vi "mudança cores.vi"() -> ()   [LabVIEW 2018]
panel:
  in  "stop":bool
  out "Thermometer":dbl(slide) scale=0.0..100.0
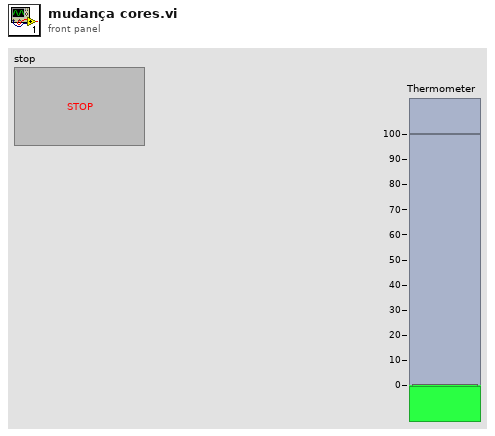
[diagram p1: front panel]
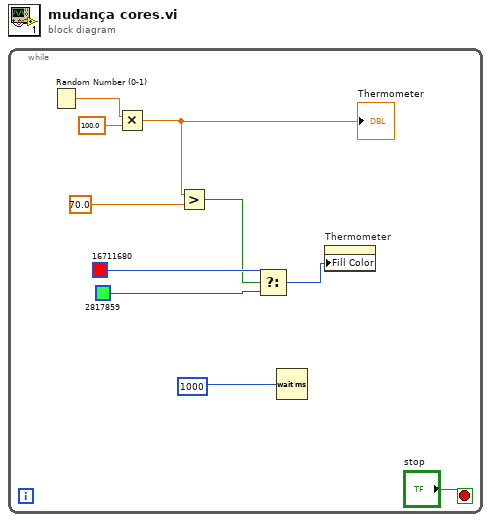
[diagram p0: block diagram]
diagram:
  n1 = while {
    stop <- "stop" stop-if-true
    n2 = Random Number (0-1)() -> (number: 0 to 1=w9:dbl)
    n3 = Multiply(x=w9, y=100.0) -> (x*y=w4:dbl)
    "Thermometer" <- w4
    n4 = Greater?(x=w4, y=70.0) -> (0:w3:bool)
    n5 = Select(t=u32 16711680, s=w3, f=u32 2817859) -> (s? t:f=w5:u32)
    n6 = Wait (ms)(milliseconds to wait=u32 1000 ("millisecond timer value")) -> ()  [unwired: 1 out]
    n7 = property on="Thermometer" class="Slide (strict)"("Fill Color"=w5) -> ()  [unwired: 2 in, 2 out]
  }
